vi "Calibrate Adjust Source.vi"(8 "error in (no error)":errorcluster, 10 "Source Value":dbl format="%#_6e", 11 "VISA resource name":refnum<visa-resource-name>="GPIB0::24::INSTR") -> (0 "error out":errorcluster, 3 "VISA resource name out":refnum<visa-resource-name>)   [LabVIEW 2022 SP3, in "Keithley 2450.lvlib"]
doc: "This VI calibrates the source function/range currently configured with the given characerized Source Value."
uses:
  Keithley 2450.lvlib
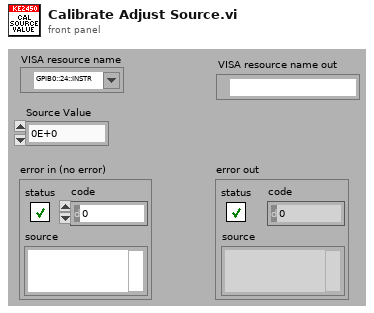
[diagram p1: front panel]
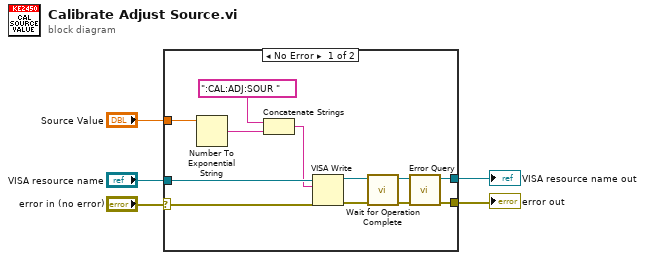
[diagram p0: block diagram]
diagram:
  n1 = case shown="No Error" "error in (no error)" {
    selector: "error in (no error)" -> [w17 w19]
    tunnel: [w11 w19] -> w4
    tunnel: "VISA resource name" -> [w16 w18]
    tunnel: [w10 w18] -> w2
    tunnel: "Source Value" -> [w12 _]
    frame No Error {
      n2 = Number To Exponential String(number=w12) -> (E-format string=w13:string)  [unwired: 3 out]
      n3 = Concatenate Strings(":CAL:ADJ:SOUR " ("string"), w13) -> (w14:string)
      n4 = VISA Write(VISA resource name=w16, write buffer=w14, error in (no error)=w17) -> (VISA resource name out=w7:refnum<visa-resource-name>, error out=w6:errorcluster)  [unwired: 1 out]
      n5 = call "Wait for Operation Complete.vi"("error in (no error)"=w6, "VISA resource name"=w7) -> ("error out"=w9:errorcluster, "VISA resource name out"=w8:refnum<visa-resource-name>)  [unwired: 8 in]
      n6 = call "Error Query.vi"("error in (no error)"=w9, "VISA resource name"=w8) -> ("error out"=w11:errorcluster, "VISA resource name out"=w10:refnum<visa-resource-name>)  [unwired: 6 in, 2 out]
    }
    frame Error {
      # "Do nothing if error condition"
    }
  }
  "error out" <- w4
  "VISA resource name out" <- w2
